vi "Verify Module is Supported.vi"(8 "error in":errorcluster, 11 "34980A in":refnum<class "34980A.lvclass">) -> (0 "error out":errorcluster, 3 "34980A out":refnum<class "34980A.lvclass">)   [LabVIEW 2019, in "34980A.lvlib" / "34980A.lvclass"]
uses:
  Library/34980A.lvclass
  Library/34980A.lvclass/34980A.ctl
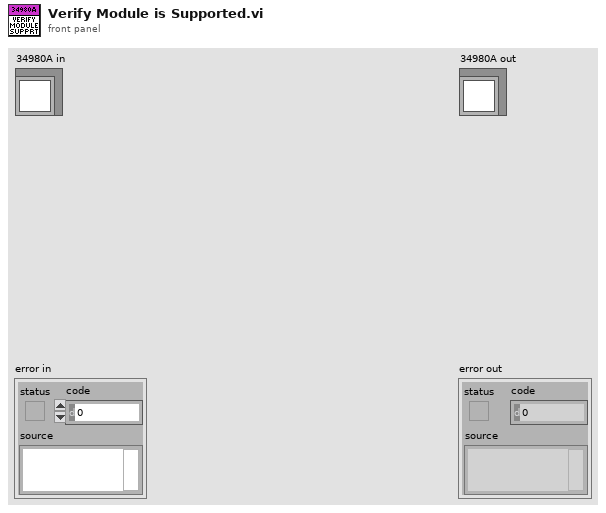
[diagram p1: front panel]
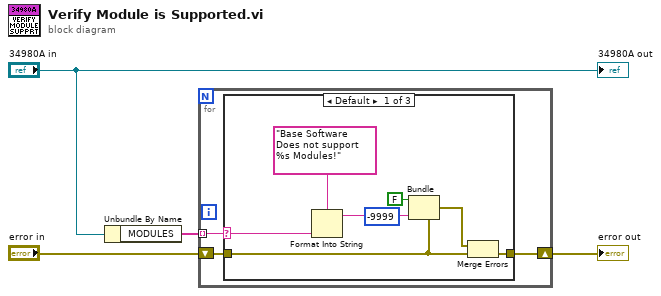
[diagram p0: block diagram]
diagram:
  n1 = Unbundle By Name("34980A in") -> ("MODULES"=w4:string[])
  n2 = for {
    tunnel: w4 -> [w6] mode=indexing
    shift-right: [w5] -> w2
    shift-left: "error in" -> [w7]
    n3 = case shown="Default" w6 {
      selector: w6 -> [w13 _ _]
      tunnel: w7 -> [w12 w16 w17]
      tunnel: [w15 w16 w17] -> w5
      frame Default {
        n4 = Format Into String(format string="Base Software Does not support %s Modules!", w13) -> (resulting string=w9:string)  [unwired: 2 in, 1 out]
        n5 = Bundle(cluster=w12, "status"=FALSE, "code"=-9999, "source"=w9) -> (w11:errorcluster)
        n6 = Merge Errors(w11, w12) -> (w15:errorcluster)
      }
      frame "34922A" {
      }
      frame "0" {
      }
    }
  }
  "error out" <- w2
  "34980A out" <- "34980A in"
